vi "read.vi"(7 "timeout (ms)":i32, 8 "error in (no error)":errorcluster, 9 "number of channels":i32, 10 "block size":i32, 11 "FPGAWrapperAN110607Galvo in":refnum<class "FPGAWrapperAN110607Galvo.lvclass">) -> (0 "error out":errorcluster, 1 "data":dbl[][](graph), 2 "FIFO full?":bool, 3 "FPGAWrapperAN110607Galvo out":refnum<class "FPGAWrapperAN110607Galvo.lvclass">, 4 "timed out?":bool)   [LabVIEW 2010, in "FPGAWrapperAN110607Galvo.lvclass"]
uses:
  FPGAWrapperAN110607Galvo.lvclass
  GenericFPGAWrapper/GenericFPGAWrapper/GenericFPGAWrapper.lvclass
  <vilib>/rvi/interface/nirviMethod/nirviMethod.xnode
  FPGA_VI_ref.ctl
  <vilib>/rvi/interface/common/niFpgaNodeNameForErrorReporting.ctl
  <vilib>/rvi/errors/niLvFpgaWhatHappensToTopLevelVI.ctl
  <vilib>/Utility/error.llb/Error Cluster From Error Code.vi
  <vilib>/rvi/errors/niLvFpgaAdjustHostInterfaceError.vi
  NiFpgaLv.dll
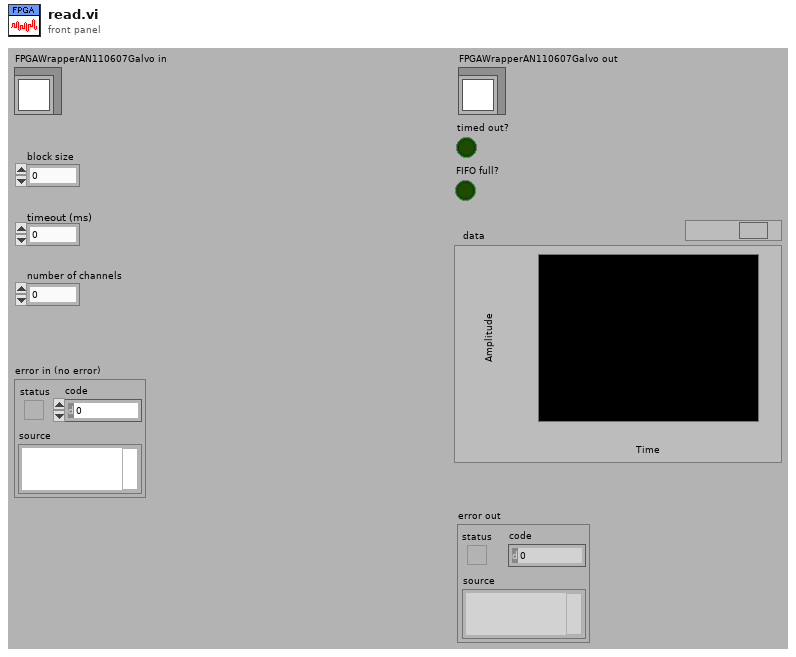
[diagram p1: front panel]
types:
  T1 = typedef "niFpgaNodeNameForErrorReporting.ctl" = enum16{"Open FPGA VI Reference", "Read/Write Control", "Invoke Method: Abort", "Invoke Method: Acknowledge IRQ", "Invoke Method: Download", "Invoke Method: FIFO.Configure", "Invoke Method: FIFO.Read", "Invoke Method: FIFO.Start", "Invoke Method: FIFO.Stop", "Invoke Method: FIFO.Write", "Invoke Method: Reset", "Invoke Method: Run", "Invoke Method: Wait on IRQ", "Close FPGA VI Reference"}
  T2 = typedef "niLvFpgaWhatHappensToTopLevelVI.ctl" = enum16{"top level VI scripted behind XNode", "top level VI inlined behind XNode"}
  T3 = typedef "FPGAWrapperAN110607Galvo.lvclass/FPGA_VI_ref.ctl" = refnum<k20>
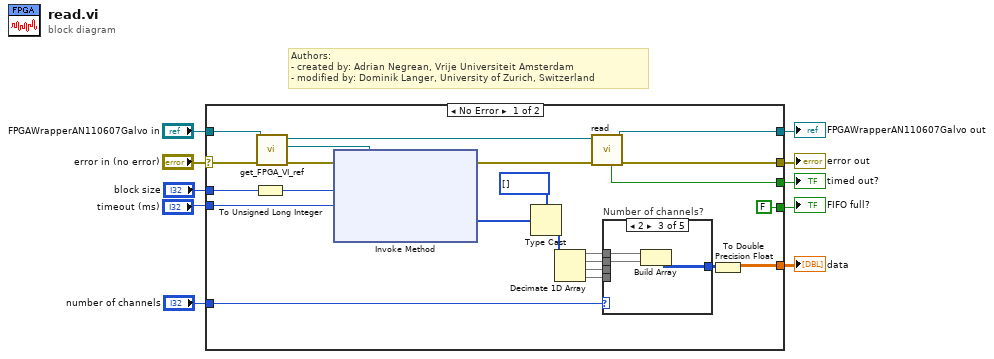
[diagram p0: block diagram]
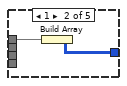
[diagram p3: hidden frame]
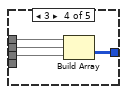
[diagram p4: hidden frame]
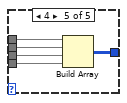
[diagram p5: hidden frame]
diagram:
  # "Authors: \n- created by: Adrian Negrean, Vrije Universiteit Amsterdam\n- modified by: Dominik Langer, University of Zurich, Switzerland"
  n1 = case shown="No Error" "error in (no error)" {
    selector: "error in (no error)" -> [w33 w122]
    tunnel: [w27 w122] -> w7
    tunnel: [w29 w121] -> w9
    tunnel: "FPGAWrapperAN110607Galvo in" -> [w32 w121]
    tunnel: "timeout (ms)" -> [w24 _]
    tunnel: "block size" -> [w31 _]
    tunnel: [w11 _] -> w4
    tunnel: [w13 _] -> w3
    tunnel: [FALSE ("FIFO full?") _] -> w2
    tunnel: "number of channels" -> [w20 _]
    frame No Error {
      n2 = To Unsigned Long Integer(number=w31) -> (unsigned 32bit integer=w25:u32)
      n3 = call-dynamic "get_FPGA_VI_ref.vi"("error in (no error)"=w33, "FPGAWrapperAN110607Galvo in"=w32) -> ("error out"=w26:errorcluster, "FPGA VI reference"=w21:T3, "FPGAWrapperAN110607Galvo out"=w30:refnum<class "FPGAWrapperAN110607Galvo.lvclass">)  [unwired: 6 in, 1 out]
      n4 = xnode "Invoke Method"("FPGA VI Reference In"=w21, "error in"=w26, "Number of Elements"=w25, "Timeout (ms)"=w24) -> ("error out"=w28:errorcluster, "Data"=w12:u64[])  [unwired: 2 out]
      n5 = Type Cast(type=u16[] [], x=w12) -> (*(type *) &x=w18:u16[])
      n6 = Decimate 1D Array(w18) -> (w17:u16[], w16:u16[], w15:u16[], w14:u16[])
      n7 = call-parent "read.vi"("error in (no error)"=w28, "GenericFPGAWrapper in"=w30) -> ("error out"=w27:errorcluster, "GenericFPGAWrapper out"=w29:refnum<class "FPGAWrapperAN110607Galvo.lvclass">, "timed out?"=w11:bool)  [unwired: 5 in, 2 out]
      n8 = case "Number of channels?" shown="2" w20 {
        tunnel: [_ w34 w36 w42 w47] -> w19
        tunnel: w17 -> [_ w35 w38 w41 w46]
        tunnel: w16 -> [_ _ w37 w40 w45]
        tunnel: w15 -> [_ _ _ w39 w44]
        tunnel: w14 -> [_ _ _ _ w43]
        frame 0, Default {
        }
        frame 1 {
          n9 = Build Array(w35) -> (w34:u16[][])
        }
        frame 2 {
          n10 = Build Array(w38, w37) -> (w36:u16[][])
        }
        frame 3 {
          n11 = Build Array(w41, w40, w39) -> (w42:u16[][])
        }
        frame 4 {
          n12 = Build Array(w46, w45, w44, w43) -> (w47:u16[][])
        }
      }
      n13 = To Double Precision Float(number=w19) -> (double precision float=w13:dbl[][])
    }
    frame Error {
    }
  }
  "error out" <- w7
  "FPGAWrapperAN110607Galvo out" <- w9
  "FIFO full?" <- w2
  "timed out?" <- w4
  "data" <- w3
